vi "FileToDoubleArray.vi"() -> (0 "Reflectance":dbl[](array[numeric]))   [LabVIEW 2013]
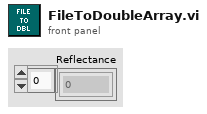
[diagram p1: front panel]
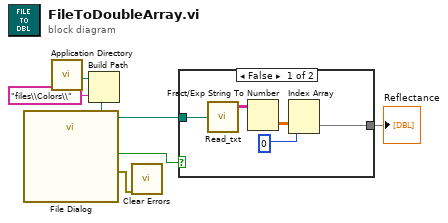
[diagram p0: block diagram]
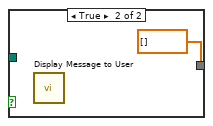
[diagram p2: hidden frame]
diagram:
  n1 = call <vilib>:"Application Directory.vi"() -> ("Application Directory"=w6:path)
  n2 = Build Path(base path=w6, name or relative path="files\\Colors\\") -> (appended path=w5:path)
  n3 = call "File Dialog"("start path"=w5) -> ("selected path"=w3:path, "cancelled"=w4:bool, "error out"=w2:errorcluster)  [unwired: 11 in, 1 out]
  n4 = call <vilib>:"Clear Errors.vi"("error in (no error)"=w2) -> ()  [unwired: 6 in, 1 out]
  n5 = case shown="False" w4 {
    tunnel: w3 -> [w9 _]
    tunnel: [w8 dbl[] []] -> w1
    frame False {
      n6 = call "Read_txt.vi"("file path (dialog if empty)"=w9) -> ("Elements"=w12:string[][])  [unwired: 2 out]
      n7 = Fract/Exp String To Number(string=w12) -> (number=w11:dbl[][])  [unwired: 3 in, 1 out]
      n8 = Index Array(array=w11, index (col)=0 ("index (row)")) -> (element=w8:dbl[])  [unwired: 1 in]
    }
    frame True {
      n9 = call "Display Message to User"() -> ()  [unwired: 10 in, 2 out]
    }
  }
  "Reflectance" <- w1
